vi "LVObject to JSON.vi"(5 "enable LabVIEW extensions? (T)":bool=TRUE, 6 "Pretty Print?":bool, 7 "Class 1 in":refnum<class "Serializer-Palette.lvclass">, 8 "error in (no error)":errorcluster, 10 "Object":refnum<class>) -> (0 "error out":errorcluster, 2 "<JSON>Object":string)   [LabVIEW 2021, in "TSC Material Theme.lvlib" / "Serializer-Palette.lvclass"]
doc: "Convert Object of a LabVIEW Class to a JSON representation."
uses:
  Serializer-Palette.lvclass
  <vilib>/JDP Science/JSONtext/LVClass Serializer/JSONtext LVClass Serializer.lvclass
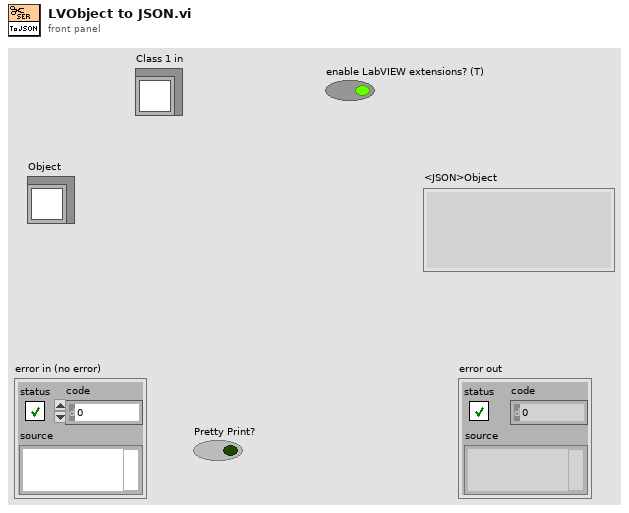
[diagram p1: front panel]
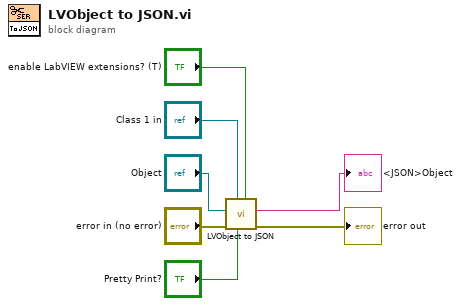
[diagram p0: block diagram]
diagram:
  n1 = call-parent "LVObject to JSON.vi"("enable LabVIEW extensions? (T)"="enable LabVIEW extensions? (T)", "Pretty Print?"="Pretty Print?", "JSONtext LVClass Serializer in"="Class 1 in", "error in (no error)"="error in (no error)", "Object"="Object") -> ("error out"=→"error out":errorcluster, "<JSON>Object"=→"<JSON>Object":string)  [unwired: 5 in]
